vi "Get Dichotomie.vi"(11 "Ball-Missile in":refnum<class "Ball-Missile.lvclass">) -> (2 "Dichotomie out":i32)   [LabVIEW 2024, in "Ball-Missile.lvclass"]
doc: "MIT Licence\nCopyright (c) 2024 David Grollier"
uses:
  Ball-Missile.lvclass
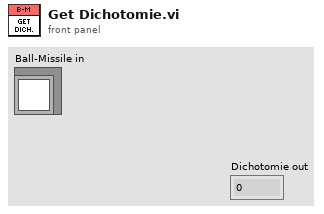
[diagram p1: front panel]
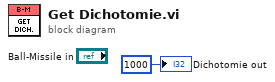
[diagram p0: block diagram]
diagram:
  "Dichotomie out" <- 1000 ("Dichotomie out")
